vi "getString.vi"(8 "error in (no error)":errorcluster, 11 "IString in":refnum<class "IString.lvclass">) -> (0 "error out":errorcluster, 2 "String out":string, 3 "IString out":refnum<class "IString.lvclass">)   [LabVIEW 2022 SP3, in "openDAQ.lvlib" / "daqCoreTypes.lvlib" / "IString.lvclass"]
uses:
  <instrlib>/openDAQ/Public/Classes/daqCoreTypes/IString/IString.lvclass
  C:/Program Files (x86)/National Instruments/LabVIEW 2022/instr.lib/openDAQ/Public/Classes/IBaseObject/IBaseObject.lvclass
  <instrlib>/openDAQ/Public/Classes/IBaseObject/IBaseObject.lvclass/IBaseObject.ctl
  <instrlib>/openDAQ/Public/Classes/IBaseObject/Accessor/Read reference.vi
  <instrlib>/openDAQ/Public/Classes/daqUtils/daqUtils.lvlib
  <instrlib>/openDAQ/Binaries/Windows/x86/copendaq32.dll
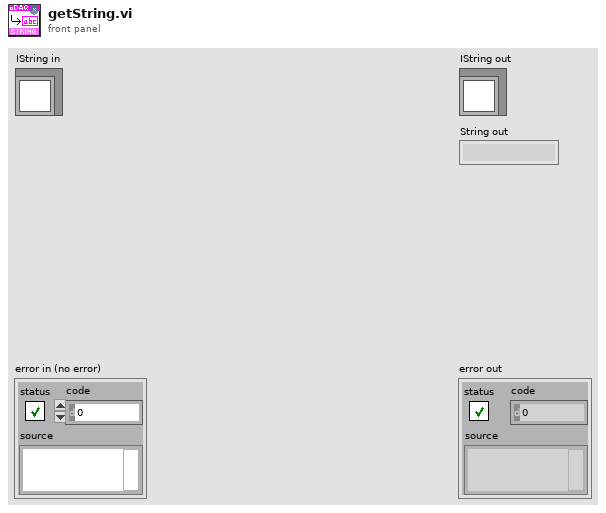
[diagram p1: front panel]
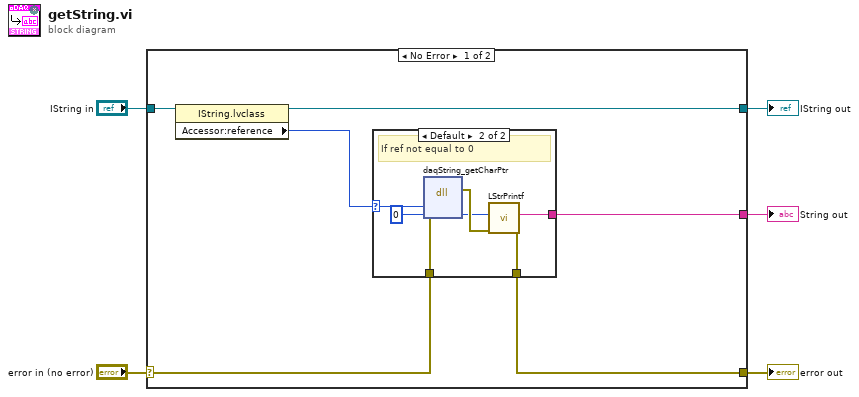
[diagram p0: block diagram]
diagram:
  n1 = case shown="No Error" "error in (no error)" {
    selector: "error in (no error)" -> [w11 w21]
    tunnel: [w9 w21] -> w4
    tunnel: [w6 w20] -> w2
    tunnel: "IString in" -> [w10 w20]
    tunnel: [w8 _] -> w1
    frame No Error {
      n2 = property class="IString.lvclass"(reference=w10) -> (reference out=w6:refnum<class "IString.lvclass">, "Accessor:reference"=w7:i64)  [unwired: 1 in, 1 out]
      n3 = case shown="Default" w7 {
        selector: w7 -> [_ w13]
        tunnel: w11 -> [w12 w18]
        tunnel: [w12 w16] -> w9
        tunnel: [_ w15] -> w8
        frame 0 {
        }
        frame Default {
          # "If ref not equal to 0"
          n4 = dll-call lib="C:/Program Files (x86)/National Instruments/LabVIEW 2022/instr.lib/openDAQ/Binaries/Windows/x86/copendaq*.*" fn="daqString_getCharPtr"(error in=w18, "daqString"=w13, "value"=i64 0) -> (error out=w19:errorcluster, "value"=w17:i64)  [unwired: 4 in, 1 out]
          n5 = call <instrlib>:"LStrPrintf.vi"("error in (no error)"=w19, "ObjectPointer"=w17) -> ("error out"=w16:errorcluster, "OutputStr"=w15:string)  [unwired: 8 in]
        }
      }
    }
    frame Error {
    }
  }
  "error out" <- w4
  "IString out" <- w2
  "String out" <- w1
